vi "createCommand.vi"(8 "error in (no error)":errorcluster, 9 "Variant":variant, 10 "Command":T1, 11 "DomeCommunicator in":refnum<class "ATDomeCommunicator.lvclass">) -> (0 "error out":errorcluster, 2 "CommandString":string, 3 "DomeCommunicator out":refnum<class "ATDomeCommunicator.lvclass">)   [LabVIEW 2016, in "ATDomeCommunicator.lvclass"]
uses:
  ATDomeCommunicator.lvclass
  ComTypedefs/commands.ctl
  IDome/domeTypedefs/azimuth.ctl
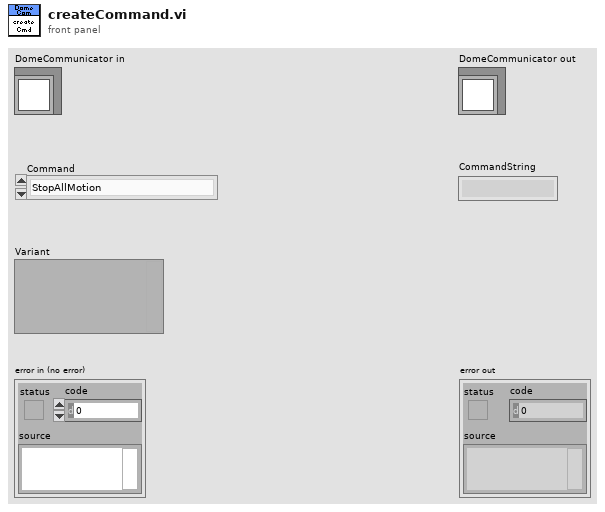
[diagram p1: front panel]
types:
  T1 = typedef "commands.ctl" = enum16{"StopAllMotion", "CloseMainDoor", "OpenMainDoor", "CloseDropoutDoor", "OpenDropoutDoor", "SynchronizedOpen", "SynchronizedClose", "AutoShutDownOn", "AutoShutDownOff", "RainOn", "RainOff", "CloudSensorOn", "CloudSensorOff", "RotateToHomePosition", "MoveToAzimuth", "SetTolerance", "DefineHomePosition", "HighSpeedThreshold", "SetCoast", "SetEncoderCountFor360", "SetWatchDogTimer", "SetReverseDirectionMotionDelay", "SaveCurrentConfiguration"}
  T2 = typedef "azimuth.ctl" = dbl
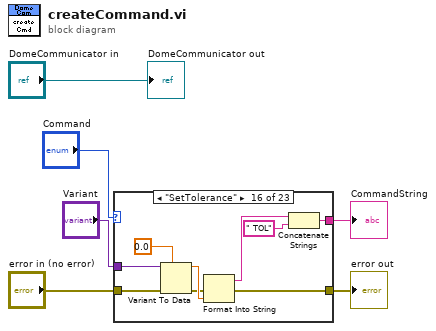
[diagram p0: block diagram]
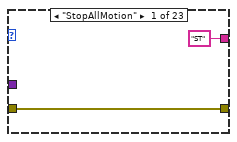
[diagram p2: hidden frame]
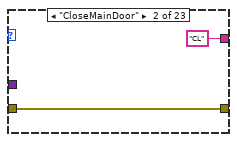
[diagram p3: hidden frame]
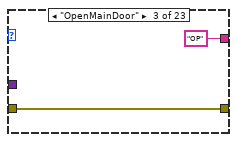
[diagram p4: hidden frame]
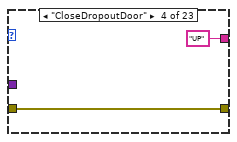
[diagram p5: hidden frame]
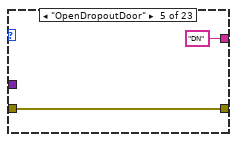
[diagram p6: hidden frame]
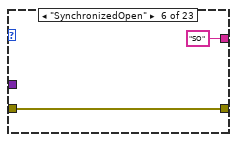
[diagram p7: hidden frame]
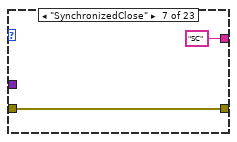
[diagram p8: hidden frame]
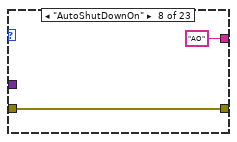
[diagram p9: hidden frame]
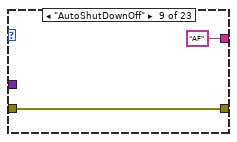
[diagram p10: hidden frame]
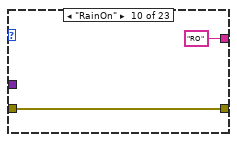
[diagram p11: hidden frame]
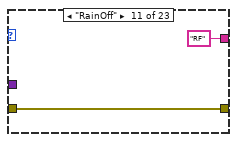
[diagram p12: hidden frame]
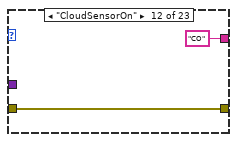
[diagram p13: hidden frame]
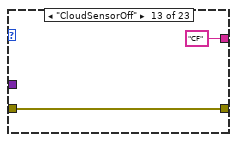
[diagram p14: hidden frame]
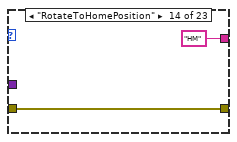
[diagram p15: hidden frame]
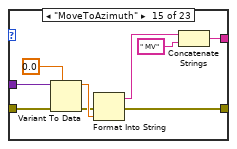
[diagram p16: hidden frame]
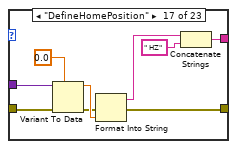
[diagram p17: hidden frame]
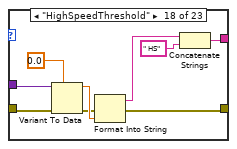
[diagram p18: hidden frame]
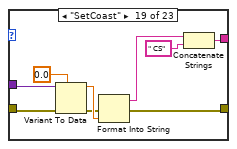
[diagram p19: hidden frame]
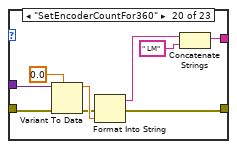
[diagram p20: hidden frame]
diagram:
  n1 = case shown="\"SetTolerance\"" "Command" {
    tunnel: ["ST" ("CommandString") "CL" ("CommandString") "OP" ("CommandString") "UP" ("CommandString") "DN" ("CommandString") "SO" ("CommandString") "SC" ("CommandString") "AO" ("CommandString") "AF" ("CommandString") "RO" ("CommandString") "RF" ("CommandString") "CO" ("CommandString") "CF" ("CommandString") "HM" ("CommandString") w40 w44 w54 w63 w72 w80 w89 w101 "CFS" ("CommandString")] -> w4
    tunnel: "Variant" -> [_ _ _ _ _ _ _ _ _ _ _ _ _ _ w43 w48 w57 w66 w74 w83 w92 w98 _]
    tunnel: "error in (no error)" -> [w7 w9 w11 w13 w15 w17 w19 w21 w23 w25 w27 w29 w31 w33 w42 w47 w56 w65 w75 w82 w91 w99 w107]
    tunnel: [w7 w9 w11 w13 w15 w17 w19 w21 w23 w25 w27 w29 w31 w33 w36 w46 w55 w64 w73 w81 w90 w100 w107] -> w1
    frame "StopAllMotion" {
    }
    frame "CloseMainDoor" {
    }
    frame "OpenMainDoor" {
    }
    frame "CloseDropoutDoor" {
    }
    frame "OpenDropoutDoor" {
    }
    frame "SynchronizedOpen" {
    }
    frame "SynchronizedClose" {
    }
    frame "AutoShutDownOn" {
    }
    frame "AutoShutDownOff" {
    }
    frame "RainOn" {
    }
    frame "RainOff" {
    }
    frame "CloudSensorOn" {
    }
    frame "CloudSensorOff" {
    }
    frame "RotateToHomePosition" {
    }
    frame "MoveToAzimuth" {
      n2 = Variant To Data(error in=w42, type=T2 0.0 ("azimuth"), Variant=w43) -> (data=w38:T2, error out=w37:errorcluster)
      n3 = Format Into String(error in=w37, w38) -> (resulting string=w35:string, error out=w36:errorcluster)  [unwired: 2 in]
      n4 = Concatenate Strings(w35, " MV" ("CommandString")) -> (w40:string)
    }
    frame "SetTolerance" {
      n5 = Variant To Data(error in=w47, type=sgl 0.0, Variant=w48) -> (data=w51:sgl, error out=w50:errorcluster)
      n6 = Format Into String(error in=w50, w51) -> (resulting string=w49:string, error out=w46:errorcluster)  [unwired: 2 in]
      n7 = Concatenate Strings(w49, " TOL" ("CommandString")) -> (w44:string)
    }
    frame "DefineHomePosition" {
      n8 = Variant To Data(error in=w56, type=T2 0.0 ("azimuth"), Variant=w57) -> (data=w60:T2, error out=w59:errorcluster)
      n9 = Format Into String(error in=w59, w60) -> (resulting string=w58:string, error out=w55:errorcluster)  [unwired: 2 in]
      n10 = Concatenate Strings(w58, " HZ" ("CommandString")) -> (w54:string)
    }
    frame "HighSpeedThreshold" {
      n11 = Variant To Data(error in=w65, type=sgl 0.0, Variant=w66) -> (data=w69:sgl, error out=w68:errorcluster)
      n12 = Format Into String(error in=w68, w69) -> (resulting string=w67:string, error out=w64:errorcluster)  [unwired: 2 in]
      n13 = Concatenate Strings(w67, " HS" ("CommandString")) -> (w63:string)
    }
    frame "SetCoast" {
      n14 = Variant To Data(error in=w75, type=sgl 0.0, Variant=w74) -> (data=w78:sgl, error out=w77:errorcluster)
      n15 = Format Into String(error in=w77, w78) -> (resulting string=w76:string, error out=w73:errorcluster)  [unwired: 2 in]
      n16 = Concatenate Strings(w76, " CS" ("CommandString")) -> (w72:string)
    }
    frame "SetEncoderCountFor360" {
      n17 = Variant To Data(error in=w82, type=sgl 0.0, Variant=w83) -> (data=w87:sgl, error out=w86:errorcluster)
      n18 = Format Into String(error in=w86, w87) -> (resulting string=w85:string, error out=w81:errorcluster)  [unwired: 2 in]
      n19 = Concatenate Strings(w85, " LM" ("CommandString")) -> (w80:string)
    }
    frame "SetWatchDogTimer" {
      n20 = Variant To Data(error in=w91, type=sgl 0.0, Variant=w92) -> (data=w96:sgl, error out=w95:errorcluster)
      n21 = Format Into String(error in=w95, w96) -> (resulting string=w94:string, error out=w90:errorcluster)  [unwired: 2 in]
      n22 = Concatenate Strings(w94, " WT" ("CommandString")) -> (w89:string)
    }
    frame "SetReverseDirectionMotionDelay" {
      n23 = Variant To Data(error in=w99, type=sgl 0.0, Variant=w98) -> (data=w105:sgl, error out=w104:errorcluster)
      n24 = Format Into String(error in=w104, w105) -> (resulting string=w103:string, error out=w100:errorcluster)  [unwired: 2 in]
      n25 = Concatenate Strings(w103, " RD" ("CommandString")) -> (w101:string)
    }
    frame "SaveCurrentConfiguration" {
    }
  }
  "error out" <- w1
  "CommandString" <- w4
  "DomeCommunicator out" <- "DomeCommunicator in"
